vi "Calculation for partial mode.vi"(0 "Глубина погружения в раствор [мм]":dbl[](array[numeric])=[20.0, 20.0, 20.0, 20.0], 1 "Опускания подложки до раствора":dbl[](array[numeric])=[2.9, 2.9, 2.9, 2.9], 2 "Опускания подложки в растворе":dbl[](array[numeric])=[1.0, 1.0, 1.0, 1.0], 3 "Подъема подложки из раствора":dbl[](array[numeric])=[1.0, 1.0, 1.0, 1.0], 4 "Подъема подложки над раствором":dbl[](array[numeric])=[2.9, 2.9, 2.9, 2.9], 5 "Steps for partial mode":dbl, 6 "Текущий раствор":i32, 8 "Нахождения в растворе":dbl[](array[numeric])=[1.0, 1.0, 1.0, 1.0] caption="Время нахождения в растворе (секунды)", 10 "Задержки после подъема из раствора":dbl[](array[numeric])=[0.0, 0.0, 0.0, 0.0]) -> (9 "Время задержки после подъема":dbl, 11 "Время нахождения в растворе":dbl, 13 "Кол-во шагов 1":dbl, 14 "Скорость 4":dbl, 15 "Скорость 3":dbl, 16 "Кол-во шагов 3":dbl, 17 "Скорость 2":dbl, 18 "Кол-во шагов 2":dbl, 19 "Скорость 1":dbl)   [LabVIEW 2016]
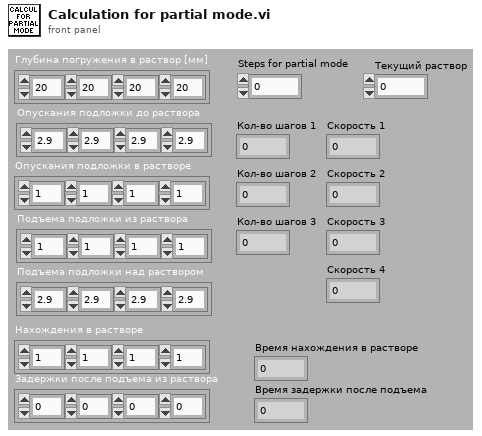
[diagram p1: front panel]
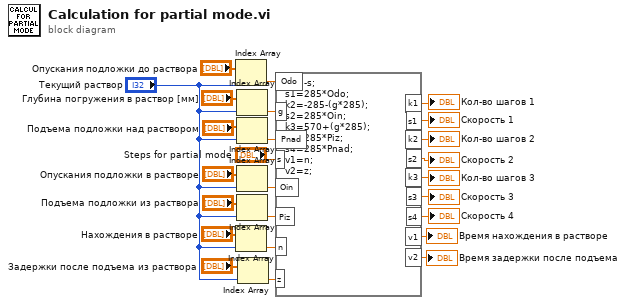
[diagram p0: block diagram]
diagram:
  n1 = Index Array(array="Опускания подложки до раствора", index="Текущий раствор") -> (element=w16:dbl)
  n2 = Index Array(array="Нахождения в растворе", index="Текущий раствор") -> (element=w6:dbl)
  n3 = Index Array(array="Глубина погружения в раствор [мм]", index="Текущий раствор") -> (element=w14:dbl)
  n4 = Index Array(array="Подъема подложки над раствором", index="Текущий раствор") -> (element=w13:dbl)
  n5 = Index Array(array="Опускания подложки в растворе", index="Текущий раствор") -> (element=w10:dbl)
  n6 = Index Array(array="Подъема подложки из раствора", index="Текущий раствор") -> (element=w9:dbl)
  n7 = Index Array(array="Задержки после подъема из раствора", index="Текущий раствор") -> (element=w7:dbl)
  n8 = formula code="k1=-s;\ns1=285*Odo;\nk2=-285-(g*285);\ns2=285*Oin;\nk3=570+(g*285);\ns3=285*Piz;\ns4=285*Pnad;\nv1=n;\nv2=z;"("Odo"=w16, "g"=w14, "Pnad"=w13, "s"="Steps for partial mode", "Oin"=w10, "Piz"=w9, "n"=w6, "z"=w7) -> ("k1"=→"Кол-во шагов 1":dbl, "s1"=→"Скорость 1":dbl, "k2"=→"Кол-во шагов 2":dbl, "s2"=→"Скорость 2":dbl, "k3"=→"Кол-во шагов 3":dbl, "s3"=→"Скорость 3":dbl, "s4"=→"Скорость 4":dbl, "v1"=→"Время нахождения в растворе":dbl, "v2"=→"Время задержки после подъема":dbl)
